vi "Solver_004.vi"(10 "Word List":string[](array[string])=["YELLOW", "ORANGE", "PURPLE", "BLUE", "GREEN", "RED"], 11 "Word Search Grid":string[][](array[string])=[["R", "B", "L", "U", "E", "W"], ["E", "G", "N", "A", "R", "O"], ["D", "B", "C", "E", "W", "L"], ["L", "L", "D", "K", "V", "L"], ["P", "U", "R", "P", "L", "E"], ["N", "E", "E", "R", "G", "Y"]]) -> (3 "Solutions":T1={"BLUE"=[{"Row"=0, "Column"=1}, {"Row"=0, "Column"=2}, {"Row"=0, "Column"=3}, {"Row"=0, "Column"=4}], "GREEN"=[{"Row"=5, "Column"=4}, {"Row"=5, "Column"=3}, {"Row"=5, "Column"=2}, {"Row"=5, "Column"=1}, {"Row"=5, "Column"=0}], "ORANGE"=[{"Row"=1, "Column"=5}, {"Row"=1, "Column"=4}, {"Row"=1, "Column"=3}, {"Row"=1, "Column"=2}, {"Row"=1, "Column"=1}, {"Row"=1, "Column"=0}], "PURPLE"=[{"Row"=4, "Column"=0}, {"Row"=4, "Column"=1}, {"Row"=4, "Column"=2}, {"Row"=4, "Column"=3}, {"Row"=4, "Column"=4}, {"Row"=4, "Column"=5}], "RED"=[{"Row"=0, "Column"=0}, {"Row"=1, "Column"=0}, {"Row"=2, "Column"=0}], "YELLOW"=[{"Row"=5, "Column"=5}, {"Row"=4, "Column"=5}, {"Row"=3, "Column"=5}, {"Row"=2, "Column"=5}, {"Row"=1, "Column"=5}, {"Row"=0, "Column"=5}]})   [LabVIEW 2022 SP3]
uses:
  Solutions--map.ctl
  Letter Index--cluster.ctl
  <vilib>/Utility/miscctls.llb/LVMapReplaceAction.ctl
panel:
  # "Do not change the connector pane of this VI."
  # "Observe the default values stored in this VI to understand how each word is represented in the Solutions map.\n\nSee the block diagram for a simple implementation of a solution. Note that this approach is not very efficient, and you will want to come up with a faster way to find the words in the grid."
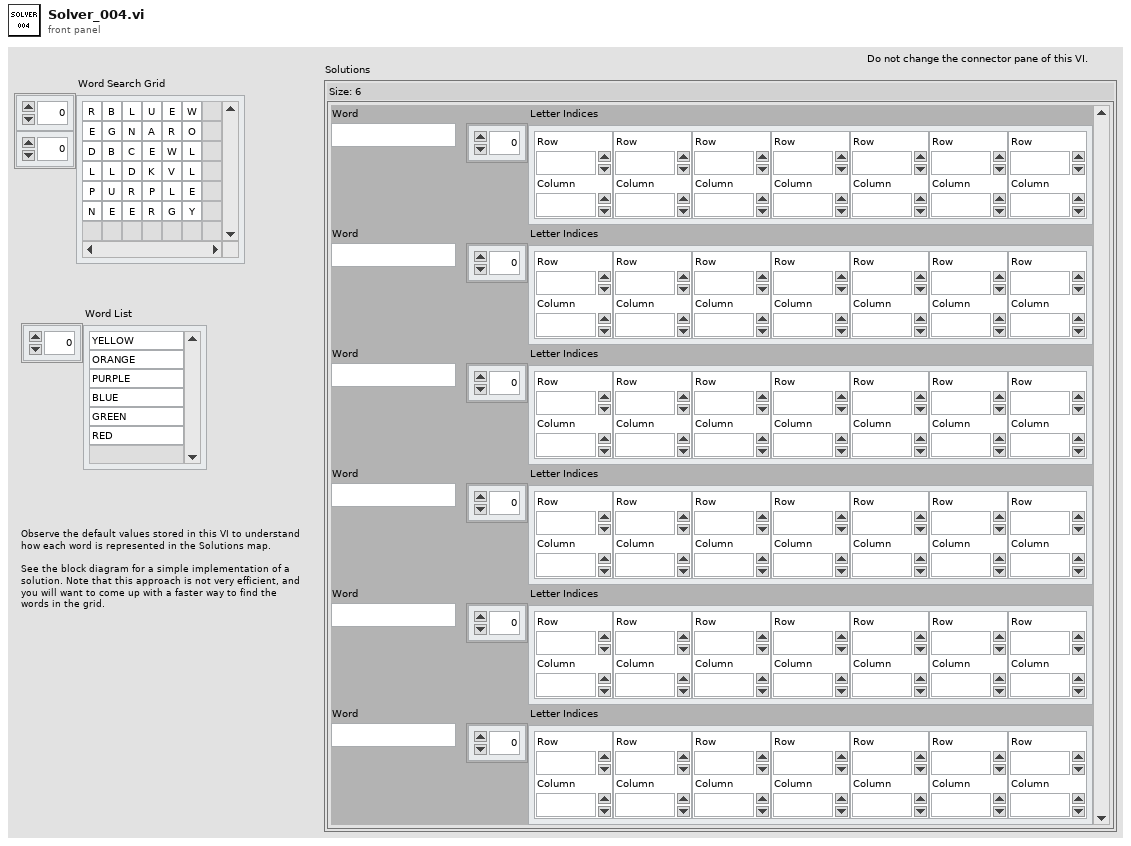
[diagram p1: front panel]
types:
  T1 = typedef "Solutions--map.ctl" = map{string, T2[]}
  T2 = typedef "Letter Index--cluster.ctl" = cluster{"Row":i32, "Column":i32}
  T3 = typedef "LVMapReplaceAction.ctl" = enum32{"Modify Entry only if found", "Add or Modify Entry", "Delete Entry"}
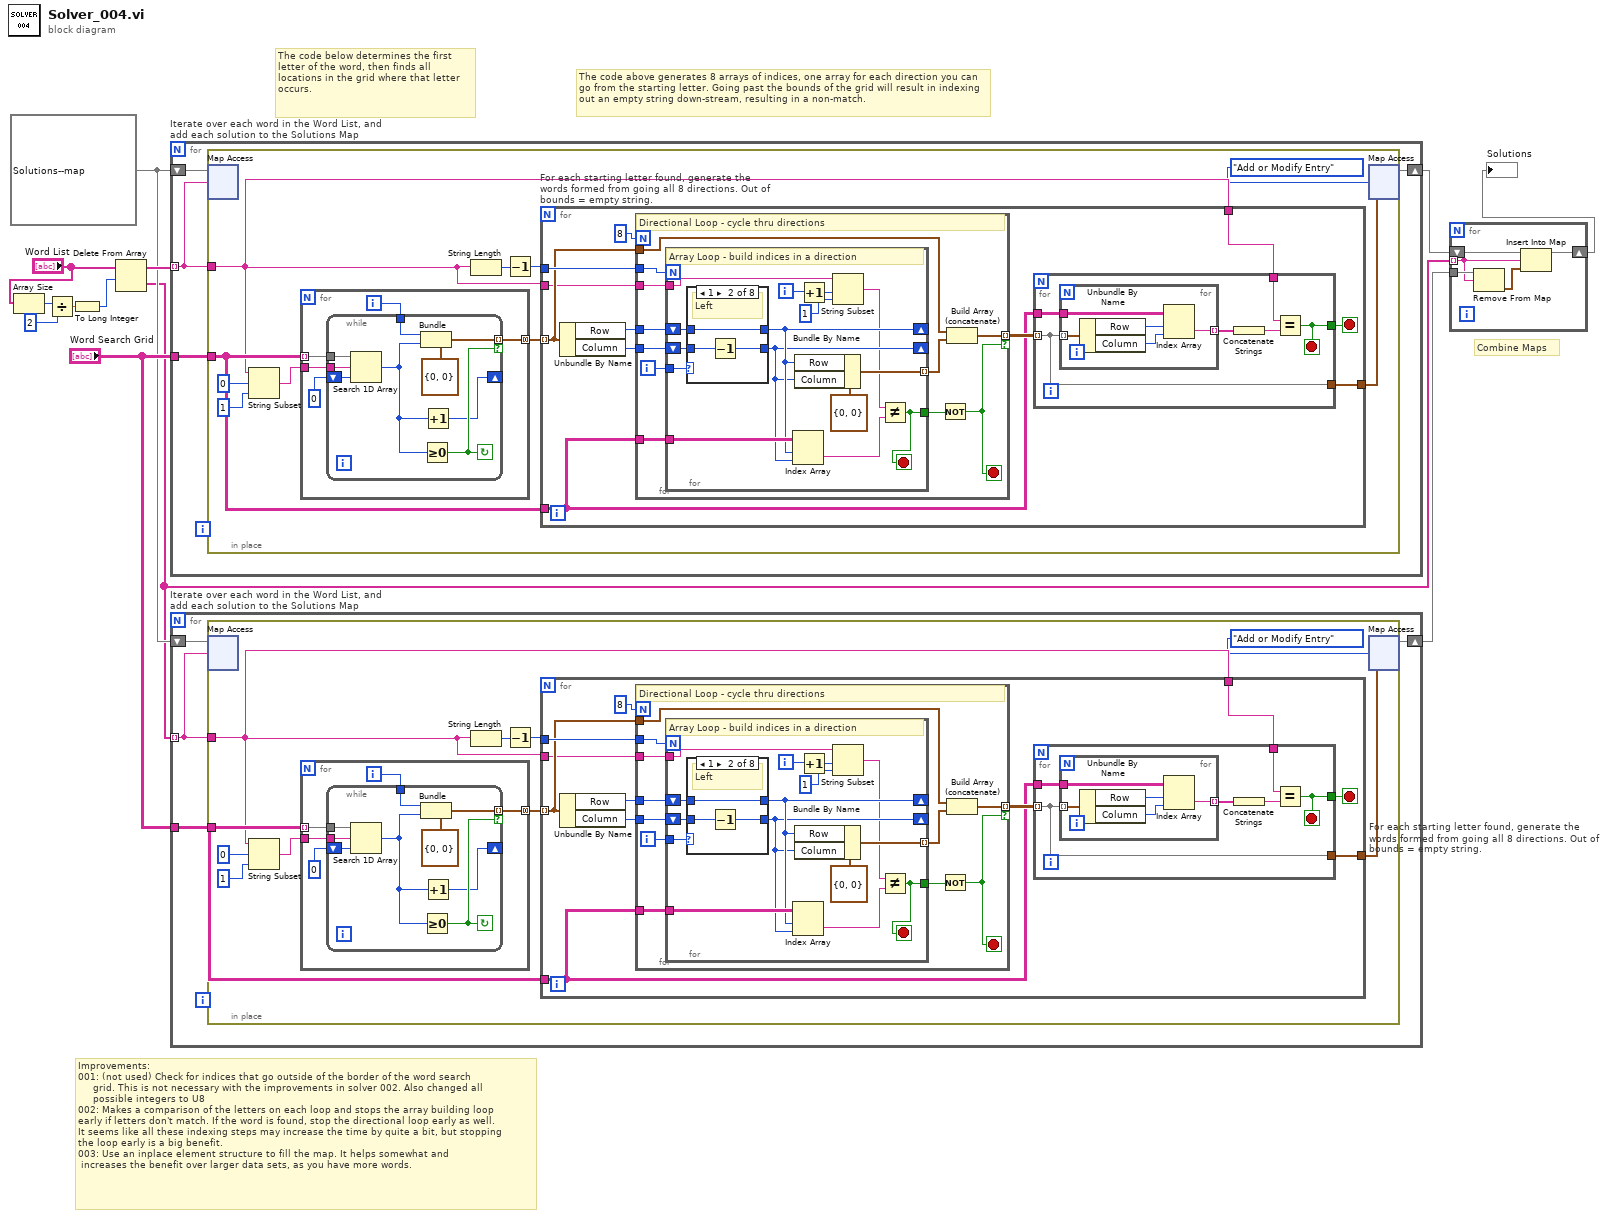
[diagram p0: block diagram]
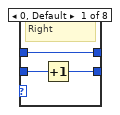
[diagram p2: hidden frame]
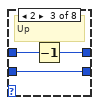
[diagram p3: hidden frame]
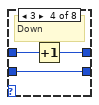
[diagram p4: hidden frame]
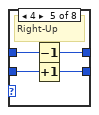
[diagram p5: hidden frame]
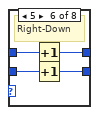
[diagram p6: hidden frame]
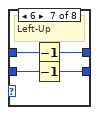
[diagram p7: hidden frame]
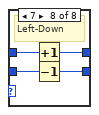
[diagram p8: hidden frame]
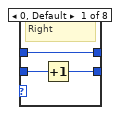
[diagram p9: hidden frame]
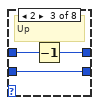
[diagram p10: hidden frame]
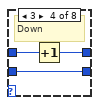
[diagram p11: hidden frame]
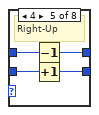
[diagram p12: hidden frame]
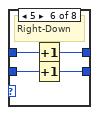
[diagram p13: hidden frame]
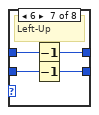
[diagram p14: hidden frame]
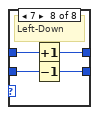
[diagram p15: hidden frame]
diagram:
  w5 = T1 {} ("Solutions")
  # "Combine Maps"
  # "The code below determines the first letter of the word, then finds all locations in the grid where that letter occurs."
  # "Improvements:\n001: (not used) Check for indices that go outside of the border of the word search\n     grid. This is not necessary with the improvements in solver 002. Also changed all \n     possible integers to U8\n002: Makes a comparison of the letters on each loop and stops the array building loop \nearly if letters don't match. If the word is found, stop the directional loop early as well. \nIt seems like all these indexing steps may increase the time by quite a bit, but stopping \nthe loop early is a big benefit.\n003: Use an inplace element structure to fill the map. It helps somewhat and \n increases the benefit over larger data sets, as you have more words."
  # "The code above generates 8 arrays of indices, one array for each direction you can go from the starting letter. Going past the bounds of the grid will result in indexing out an empty string down-stream, resulting in a non-match."
  n1 = Array Size(array="Word List") -> (size(s)=w11:i32)
  n2 = Divide(x=w11, y=2) -> (x/y=w9:dbl)
  n3 = To Long Integer(number=w9) -> (32bit integer=w8:i32)
  n4 = Delete From Array(array="Word List", length=w8) -> (deleted portion=w4:string[], array with subset deleted=w7:string[])  [unwired: 1 in]
  n5 = for "Iterate over each word in the Word List, and add each solution to the Solutions Map" {
    tunnel: "Word Search Grid" -> [w16]
    tunnel: w7 -> [w14] mode=indexing
    shift-right: [w13] -> w2
    shift-left: w5 -> [w15]
    n6 = in-place {
      in-place-border: w16 -> [w20]
      in-place-border: w14 -> [w19]
      n7 = in-place-map #1(w15, w14) -> ()  [unwired: 1 in, 2 out]
      n8 = String Subset(string=w19, offset (0)=u8 0, length (rest)=u8 1 ("length (rest)")) -> (substring=w25:string)
      n9 = for {
        tunnel: w20 -> [w107] mode=indexing
        tunnel: w25 -> [w106]
        tunnel: [w104] -> w24 mode=concatenating
        i -> [w105]
        n10 = while {
          tunnel: w107 -> [w116]
          tunnel: w106 -> [w115]
          tunnel: w105 -> [w113]
          tunnel: [w112] -> w104 mode=indexing if=w111
          shift-right: [w108] -> _
          shift-left: 0 -> [w110]
          stop <- w111 continue-if-true
          n11 = Search 1D Array(1D array=w116, element=w115, start index (0)=w110) -> (index of element=w109:i32)
          n12 = Bundle(cluster=T2 {"Row"=0, "Column"=0} ("Letter Index"), "Row"=w113, "Column"=w109) -> (w112:T2)
          n13 = Greater Or Equal To 0?(x=w109) -> (x >= 0?=w111:bool)
          n14 = Increment(x=w109) -> (x+1=w108:i32)
        }
      }
      n15 = String Length(string=w19) -> (length=w22:i32)
      n16 = Decrement(x=w22) -> (x-1=w21:i32)
      n17 = for "For each starting letter found, generate the words formed from going all 8 directions. Out of bounds = empty string." {
        tunnel: w24 -> [w33] mode=indexing
        tunnel: w21 -> [w36]
        tunnel: w20 -> [w27]
        tunnel: [w31] -> w18
        tunnel: w19 -> [w30]
        tunnel: w19 -> [w28]
        stop <- w29 stop-if-true
        n18 = Unbundle By Name(w33) -> ("Row"=w35:i32, "Column"=w34:i32)
        n19 = for {
          N: 8 -> [_]
          tunnel: w36 -> [w59]
          tunnel: w35 -> [w58]
          tunnel: w34 -> [w57]
          tunnel: w33 -> [w54]
          tunnel: [w53] -> w32 mode=indexing if=w49
          tunnel: w28 -> [w52]
          tunnel: w27 -> [w51]
          i -> [w56]
          stop <- w49 stop-if-true
          # "Directional Loop - cycle thru directions"
          n20 = for {
            N: w59 -> [_]
            tunnel: w56 -> [w72]
            tunnel: [w70] -> w55 mode=indexing
            shift-right: [w66] -> _
            shift-left: w58 -> [w74]
            shift-right: [w65] -> _
            shift-left: w57 -> [w73]
            tunnel: [w60] -> w50
            tunnel: w52 -> [w68]
            tunnel: w51 -> [w67]
            i -> [w64]
            stop <- w60 stop-if-true
            # "Array Loop - build indices in a direction"
            n21 = case shown="1" w72 {
              tunnel: w74 -> [w75 w78 w82 w85 w89 w93 w97 w101]
              tunnel: w73 -> [w77 w80 w83 w86 w90 w94 w98 w102]
              tunnel: [w76 w79 w83 w86 w87 w91 w95 w99] -> w65
              tunnel: [w75 w78 w81 w84 w88 w92 w96 w100] -> w66
              frame 0, Default {
                # "Right"
                n22 = Increment(x=w77) -> (x+1=w76:i32)
              }
              frame 1 {
                # "Left"
                n23 = Decrement(x=w80) -> (x-1=w79:i32)
              }
              frame 2 {
                # "Up"
                n24 = Decrement(x=w82) -> (x-1=w81:i32)
              }
              frame 3 {
                # "Down"
                n25 = Increment(x=w85) -> (x+1=w84:i32)
              }
              frame 4 {
                # "Right-Up"
                n26 = Decrement(x=w89) -> (x-1=w88:i32)
                n27 = Increment(x=w90) -> (x+1=w87:i32)
              }
              frame 5 {
                # "Right-Down"
                n28 = Increment(x=w93) -> (x+1=w92:i32)
                n29 = Increment(x=w94) -> (x+1=w91:i32)
              }
              frame 6 {
                # "Left-Up"
                n30 = Decrement(x=w97) -> (x-1=w96:i32)
                n31 = Decrement(x=w98) -> (x-1=w95:i32)
              }
              frame 7 {
                # "Left-Down"
                n32 = Increment(x=w101) -> (x+1=w100:i32)
                n33 = Decrement(x=w102) -> (x-1=w99:i32)
              }
            }
            n34 = Index Array(array=w67, index (row)=w66, index (col)=w65) -> (element=w62:string)
            n35 = Bundle By Name(cluster=T2 {"Row"=0, "Column"=0} ("Letter Index"), "Row"=w66, "Column"=w65) -> (w70:T2)
            n36 = Increment(x=w64) -> (x+1=w63:i32)
            n37 = String Subset(string=w68, offset (0)=w63, length (rest)=1 ("length (rest)")) -> (substring=w61:string)
            n38 = Not Equal?(x=w61, y=w62) -> (x != y?=w60:bool)
          }
          n39 = Not(x=w50) -> (.not. x?=w49:bool)
          n40 = Build Array (concatenate)(w54, w55) -> (w53:T2[])
        }
        n41 = for {
          tunnel: w32 -> [w40] mode=indexing
          tunnel: w27 -> [w43]
          tunnel: [w40] -> w31
          tunnel: w30 -> [w39]
          tunnel: [w38] -> w29
          stop <- w38 stop-if-true
          n42 = for {
            tunnel: w40 -> [w48] mode=indexing
            tunnel: w43 -> [w46]
            tunnel: [w44] -> w42 mode=indexing
            n43 = Unbundle By Name(w48) -> ("Row"=w47:i32, "Column"=w45:i32)
            n44 = Index Array(array=w46, index (row)=w47, index (col)=w45) -> (element=w44:string)
          }
          n45 = Concatenate Strings(w42) -> (w41:string)
          n46 = Equal?(x=w39, y=w41) -> (x = y?=w38:bool)
        }
      }
      n47 = in-place-map #1(w18, LVMapReplaceAction."Add or Modify Entry" ("action")) -> (w13:T1)  [unwired: 2 out]
    }
  }
  n48 = for "Iterate over each word in the Word List, and add each solution to the Solutions Map" {
    tunnel: "Word Search Grid" -> [w120]
    tunnel: w4 -> [w118] mode=indexing
    shift-right: [w117] -> w3
    shift-left: w5 -> [w119]
    n49 = in-place {
      in-place-border: w120 -> [w124]
      in-place-border: w118 -> [w123]
      n50 = in-place-map #2(w119, w118) -> ()  [unwired: 1 in, 2 out]
      n51 = String Subset(string=w123, offset (0)=u8 0, length (rest)=u8 1 ("length (rest)")) -> (substring=w129:string)
      n52 = for {
        tunnel: w124 -> [w211] mode=indexing
        tunnel: w129 -> [w210]
        tunnel: [w208] -> w128 mode=concatenating
        i -> [w209]
        n53 = while {
          tunnel: w211 -> [w220]
          tunnel: w210 -> [w219]
          tunnel: w209 -> [w217]
          tunnel: [w216] -> w208 mode=indexing if=w215
          shift-right: [w212] -> _
          shift-left: 0 -> [w214]
          stop <- w215 continue-if-true
          n54 = Search 1D Array(1D array=w220, element=w219, start index (0)=w214) -> (index of element=w213:i32)
          n55 = Bundle(cluster=T2 {"Row"=0, "Column"=0} ("Letter Index"), "Row"=w217, "Column"=w213) -> (w216:T2)
          n56 = Greater Or Equal To 0?(x=w213) -> (x >= 0?=w215:bool)
          n57 = Increment(x=w213) -> (x+1=w212:i32)
        }
      }
      n58 = String Length(string=w123) -> (length=w126:i32)
      n59 = Decrement(x=w126) -> (x-1=w125:i32)
      n60 = for "For each starting letter found, generate the words formed from going all 8 directions. Out of bounds = empty string." {
        tunnel: w128 -> [w137] mode=indexing
        tunnel: w125 -> [w140]
        tunnel: w124 -> [w131]
        tunnel: [w135] -> w122
        tunnel: w123 -> [w134]
        tunnel: w123 -> [w132]
        stop <- w133 stop-if-true
        n61 = Unbundle By Name(w137) -> ("Row"=w139:i32, "Column"=w138:i32)
        n62 = for {
          N: 8 -> [_]
          tunnel: w140 -> [w163]
          tunnel: w139 -> [w162]
          tunnel: w138 -> [w161]
          tunnel: w137 -> [w158]
          tunnel: [w157] -> w136 mode=indexing if=w153
          tunnel: w132 -> [w156]
          tunnel: w131 -> [w155]
          i -> [w160]
          stop <- w153 stop-if-true
          # "Directional Loop - cycle thru directions"
          n63 = for {
            N: w163 -> [_]
            tunnel: w160 -> [w176]
            tunnel: [w174] -> w159 mode=indexing
            shift-right: [w170] -> _
            shift-left: w162 -> [w178]
            shift-right: [w169] -> _
            shift-left: w161 -> [w177]
            tunnel: [w164] -> w154
            tunnel: w156 -> [w172]
            tunnel: w155 -> [w171]
            i -> [w168]
            stop <- w164 stop-if-true
            # "Array Loop - build indices in a direction"
            n64 = case shown="1" w176 {
              tunnel: w178 -> [w179 w182 w186 w189 w193 w197 w201 w205]
              tunnel: w177 -> [w181 w184 w187 w190 w194 w198 w202 w206]
              tunnel: [w180 w183 w187 w190 w191 w195 w199 w203] -> w169
              tunnel: [w179 w182 w185 w188 w192 w196 w200 w204] -> w170
              frame 0, Default {
                # "Right"
                n65 = Increment(x=w181) -> (x+1=w180:i32)
              }
              frame 1 {
                # "Left"
                n66 = Decrement(x=w184) -> (x-1=w183:i32)
              }
              frame 2 {
                # "Up"
                n67 = Decrement(x=w186) -> (x-1=w185:i32)
              }
              frame 3 {
                # "Down"
                n68 = Increment(x=w189) -> (x+1=w188:i32)
              }
              frame 4 {
                # "Right-Up"
                n69 = Decrement(x=w193) -> (x-1=w192:i32)
                n70 = Increment(x=w194) -> (x+1=w191:i32)
              }
              frame 5 {
                # "Right-Down"
                n71 = Increment(x=w197) -> (x+1=w196:i32)
                n72 = Increment(x=w198) -> (x+1=w195:i32)
              }
              frame 6 {
                # "Left-Up"
                n73 = Decrement(x=w201) -> (x-1=w200:i32)
                n74 = Decrement(x=w202) -> (x-1=w199:i32)
              }
              frame 7 {
                # "Left-Down"
                n75 = Increment(x=w205) -> (x+1=w204:i32)
                n76 = Decrement(x=w206) -> (x-1=w203:i32)
              }
            }
            n77 = Index Array(array=w171, index (row)=w170, index (col)=w169) -> (element=w166:string)
            n78 = Bundle By Name(cluster=T2 {"Row"=0, "Column"=0} ("Letter Index"), "Row"=w170, "Column"=w169) -> (w174:T2)
            n79 = Increment(x=w168) -> (x+1=w167:i32)
            n80 = String Subset(string=w172, offset (0)=w167, length (rest)=1 ("length (rest)")) -> (substring=w165:string)
            n81 = Not Equal?(x=w165, y=w166) -> (x != y?=w164:bool)
          }
          n82 = Not(x=w154) -> (.not. x?=w153:bool)
          n83 = Build Array (concatenate)(w158, w159) -> (w157:T2[])
        }
        n84 = for {
          tunnel: w136 -> [w144] mode=indexing
          tunnel: w131 -> [w147]
          tunnel: [w144] -> w135
          tunnel: w134 -> [w143]
          tunnel: [w142] -> w133
          stop <- w142 stop-if-true
          n85 = for {
            tunnel: w144 -> [w152] mode=indexing
            tunnel: w147 -> [w150]
            tunnel: [w148] -> w146 mode=indexing
            n86 = Unbundle By Name(w152) -> ("Row"=w151:i32, "Column"=w149:i32)
            n87 = Index Array(array=w150, index (row)=w151, index (col)=w149) -> (element=w148:string)
          }
          n88 = Concatenate Strings(w146) -> (w145:string)
          n89 = Equal?(x=w143, y=w145) -> (x = y?=w142:bool)
        }
      }
      n90 = in-place-map #2(w122, LVMapReplaceAction."Add or Modify Entry" ("action")) -> (w117:T1)  [unwired: 2 out]
    }
  }
  n91 = for {
    tunnel: w4 -> [w222] mode=indexing
    tunnel: w3 -> [w225]
    shift-right: [w221] -> w1
    shift-left: w2 -> [w224]
    n92 = Remove From Map(10:w222, 11:w225) -> (1:w223:T2[])  [unwired: 2 out]
    n93 = Insert Into Map(map in=w224, key=w222, value=w223) -> (map out=w221:T1)  [unwired: 2 out]
  }
  "Solutions" <- w1
